vi "Read Waveform (Voltage).vi"(0 "VISA resource name":refnum<visa-resource-name>, 11 "error in (no error)":errorcluster) -> (4 "VISA resource name out":refnum<visa-resource-name>, 6 "Waveform (V)":waveform(dbl), 15 "error out":errorcluster)   [LabVIEW 2020, in "NH Research Regenerative Test Series.lvlib"]
doc: "Initiates a measurement and returns a waveform containing the instantaneous input voltage in Volts. Query Number of Samples is called internally after the measurement has been initiated to read how many samples are available to read from the instruments buffer.\n\nWaveforms are captured with every initiated measurement based on the Set Aperture Length.vi and Set Number of Samples.vi commands. A measurement must be initiated first using a Read command or calling Initiate Measurement.vi."
uses:
  NH Research Regenerative Test Series.lvlib
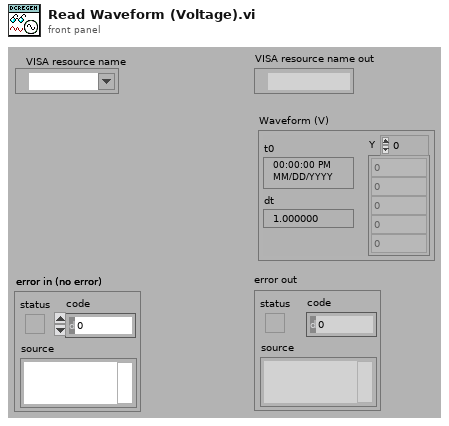
[diagram p1: front panel]
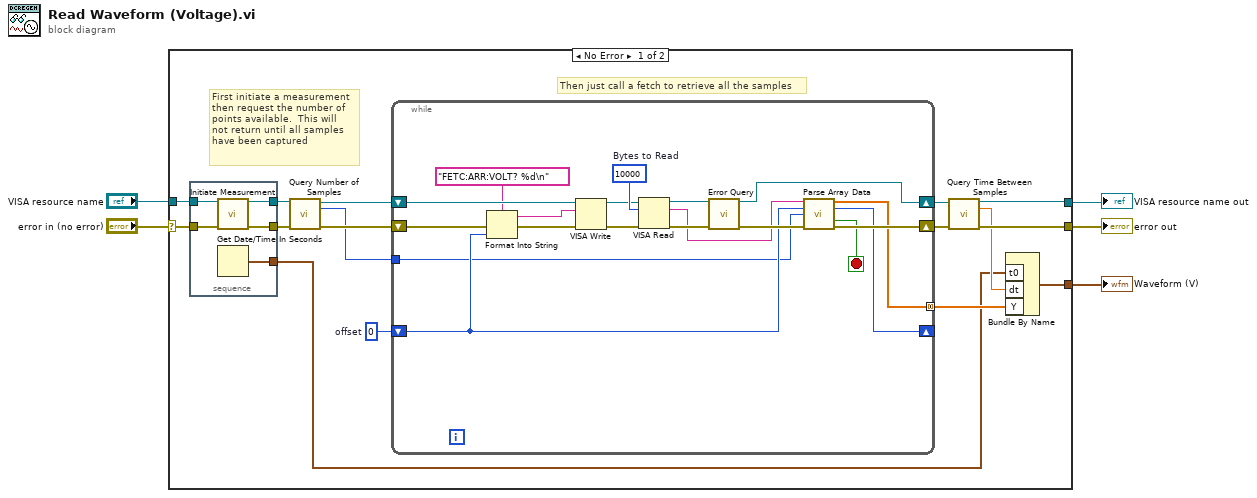
[diagram p0: block diagram]
diagram:
  n1 = case shown="No Error" "error in (no error)" {
    selector: "error in (no error)" -> [w10 w47]
    tunnel: [w14 w47] -> w4
    tunnel: [w11 w46] -> w2
    tunnel: "VISA resource name" -> [w9 w46]
    tunnel: [w12 _] -> w1
    frame No Error {
      w21 = 0  # offset
      # "Then just call a fetch to retrieve all the samples"
      # "First initiate a measurement\nthen request the number of\npoints available.  This will\nnot return until all samples\nhave been captured"
      n2 = stacked-sequence {
        tunnel: w10 -> [w26]
        tunnel: w9 -> [w25]
        tunnel: [w24] -> w8
        tunnel: [w23] -> w7
        tunnel: [w22] -> w6
        frame #0 {
          n3 = call "Initiate Measurement.vi"("VISA resource name"=w25, "error in (no error)"=w26) -> ("VISA resource name out"=w23:refnum<visa-resource-name>, "error out"=w24:errorcluster)  [unwired: 12 in]
          n4 = Get Date/Time In Seconds() -> (seconds since 1Jan1904=w22:timestamp)
        }
      }
      n5 = call "Query Number of Samples.vi"("VISA resource name"=w7, "error in (no error)"=w8) -> ("VISA resource name out"=w20:refnum<visa-resource-name>, "Number of Samples"=w18:u32, "error out"=w19:errorcluster)  [unwired: 11 in]
      n6 = while {
        shift-right: [w34] -> w16
        shift-left: w19 -> [w38]
        shift-right: [w27] -> w17
        shift-left: w20 -> [w42]
        tunnel: [w29] -> w15 mode=concatenating
        shift-right: [w30] -> _
        shift-left: w21 -> [w32]
        tunnel: w18 -> [w31]
        stop <- w28 stop-if-true
        w45 = u32 10000  # Bytes to Read
        n7 = Format Into String(format string="FETC:ARR:VOLT? %d\n", error in=w38, w32) -> (resulting string=w36:string, error out=w37:errorcluster)  [unwired: 1 in]
        n8 = VISA Write(VISA resource name=w42, write buffer=w36, error in (no error)=w37) -> (VISA resource name out=w43:refnum<visa-resource-name>, error out=w44:errorcluster)  [unwired: 1 out]
        n9 = VISA Read(VISA resource name=w43, byte count=w45, error in (no error)=w44) -> (VISA resource name out=w41:refnum<visa-resource-name>, read buffer=w33:string, error out=w40:errorcluster)  [unwired: 1 out]
        n10 = call "Error Query.vi"("VISA resource name"=w41, "error in (no error)"=w40) -> ("VISA resource name out"=w27:refnum<visa-resource-name>, "error out"=w35:errorcluster)  [unwired: 10 in, 2 out]
        n11 = call "Parse Array Data.vi"("Samples String"=w33, "Current Index"=w32, "Number of Samples"=w31, "error in (no error)"=w35) -> ("Samples"=w29:dbl[], "Next Index"=w30:i32, "Stop Reading Samples"=w28:bool, "error out"=w34:errorcluster)  [unwired: 8 in]
      }
      n12 = call "Query Time Between Samples.vi"("VISA resource name"=w17, "error in (no error)"=w16) -> ("VISA resource name out"=w11:refnum<visa-resource-name>, "Time Interval (s)"=w13:dbl, "error out"=w14:errorcluster)  [unwired: 11 in]
      n13 = Bundle By Name("t0"=w6, "dt"=w13, "Y"=w15) -> (w12:waveform(dbl))  [unwired: 1 in]
    }
    frame Error {
    }
  }
  "error out" <- w4
  "VISA resource name out" <- w2
  "Waveform (V)" <- w1
